vi "cREATE.vi"(8 "error in (no error)":errorcluster) -> (0 "error out":errorcluster, 3 "FIFO class out":refnum<class "FIFO class.lvclass">)   [LabVIEW 2021, in "RT Classes.lvlib" / "FIFO class.lvclass"]
uses:
  FIFO class.lvclass
  FIFO class.lvclass/FIFO class.ctl
  <vilib>/FPGAPlugInAG/myRIO-1900/niLvFpga_Open_myRIO-1900.vi
  <vilib>/rvi/interface/common/dynamic/niFpgaDynamicAddResources.vi
  <vilib>/Utility/error.llb/Error Cluster From Error Code.vi
  <vilib>/rvi/interface/nirviOpenFPGA/nirviOpenFPGA.xnode
  FPGA Bitfiles/lightstripprojec_FPGATarget_FPGAMain_V6m3OHc8nzM.lvbitx
  FPGA Main.vi
  <vilib>/rvi/interface/nirviMethod/nirviMethod.xnode
  <vilib>/FPGAPlugInAG/Dynamic/niLvFpga_StartFifo_Dynamic.vi
  <vilib>/rvi/errors/niLvFpgaMergeErrorWithErrorCode.vi
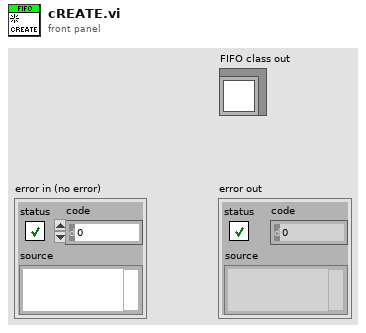
[diagram p1: front panel]
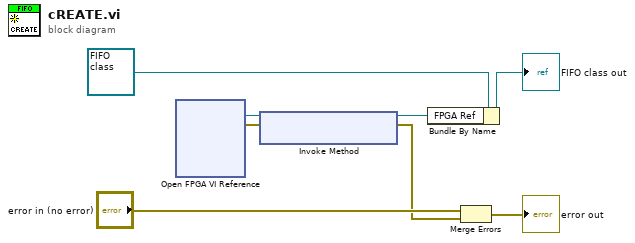
[diagram p0: block diagram]
diagram:
  n1 = xnode "Open FPGA VI Reference"() -> ("FPGA VI Reference Out"=w6:refnum<k20>, "error out"=w5:errorcluster)  [unwired: 2 in]
  n2 = xnode "Invoke Method"("FPGA VI Reference In"=w6, "error in"=w5) -> ("FPGA VI Reference Out"=w3:refnum<k20>, "error out"=w1:errorcluster)
  n3 = Bundle By Name(cluster=refnum<class "FIFO class.lvclass"> refnum ("FIFO class in"), "FPGA Ref"=w3) -> (→"FIFO class out":refnum<class "FIFO class.lvclass">)
  n4 = Merge Errors("error in (no error)", w1) -> (→"error out":errorcluster)
